vi "SRS Lockin Get Range.vi"(8 "error in (no error)":errorcluster, 11 "VISA resource name":refnum<visa-resource-name>) -> (0 "error out":errorcluster, 3 "VISA resource name out":refnum<visa-resource-name>, 5 "Range, V":sgl format="%#_6e")   [LabVIEW 2015]
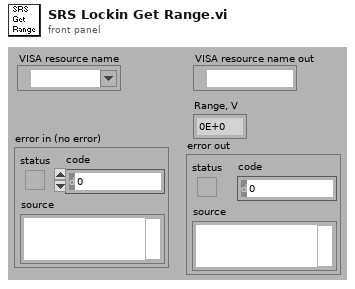
[diagram p1: front panel]
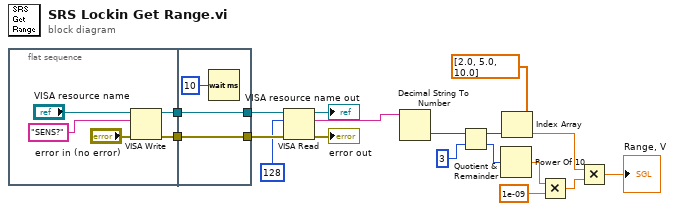
[diagram p0: block diagram]
diagram:
  n1 = flat-sequence {
    tunnel: [w23] -> w2
    tunnel: [w22] -> w1
    tunnel: [w25] -> w16
    tunnel: [w26] -> w17
    tunnel: w2 -> [w26]
    tunnel: w1 -> [w25]
    frame #0 {
      n2 = VISA Write(VISA resource name="VISA resource name", write buffer="SENS?", error in (no error)="error in (no error)") -> (VISA resource name out=w22:refnum<visa-resource-name>, error out=w23:errorcluster)  [unwired: 1 out]
    }
    frame #1 {
      n3 = Wait (ms)(milliseconds to wait=u32 10) -> ()  [unwired: 1 out]
    }
  }
  n4 = VISA Read(VISA resource name=w16, byte count=u32 128, error in (no error)=w17) -> (VISA resource name out=→"VISA resource name out":refnum<visa-resource-name>, read buffer=w18:string, error out=→"error out":errorcluster)  [unwired: 1 out]
  n5 = Decimal String To Number(string=w18) -> (number=w13:i32)  [unwired: 3 out]
  n6 = Quotient & Remainder(x=w13, y=3) -> (x-y*floor(x/y)=w10:i32, floor(x/y)=w9:i32)
  n7 = Power Of 10(x=w9) -> (10^x=w8:dbl)
  n8 = Index Array(array=dbl[] [2.0, 5.0, 10.0], index=w10) -> (element=w4:dbl)
  n9 = Multiply(x=w8, y=1e-09) -> (x*y=w5:dbl)
  n10 = Multiply(x=w4, y=w5) -> (x*y=→"Range, V":dbl)
